vi "Unescape JSON String.vi"(11 "escaped string":string) -> (3 "regular string":string)   [LabVIEW 2020, in "Multi Error Cluster.lvlib"]
doc: "Convert an escaped JSON stringh into the originally supplied string. This allows a name to contain a /, '\", \\, or a control character."
uses:
  <vilib>/MultiError/TokenizeJSON/Multi Error Cluster.lvlib
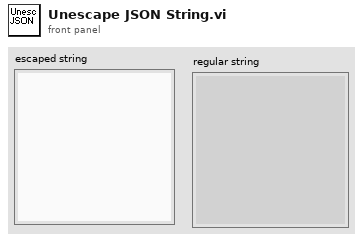
[diagram p1: front panel]
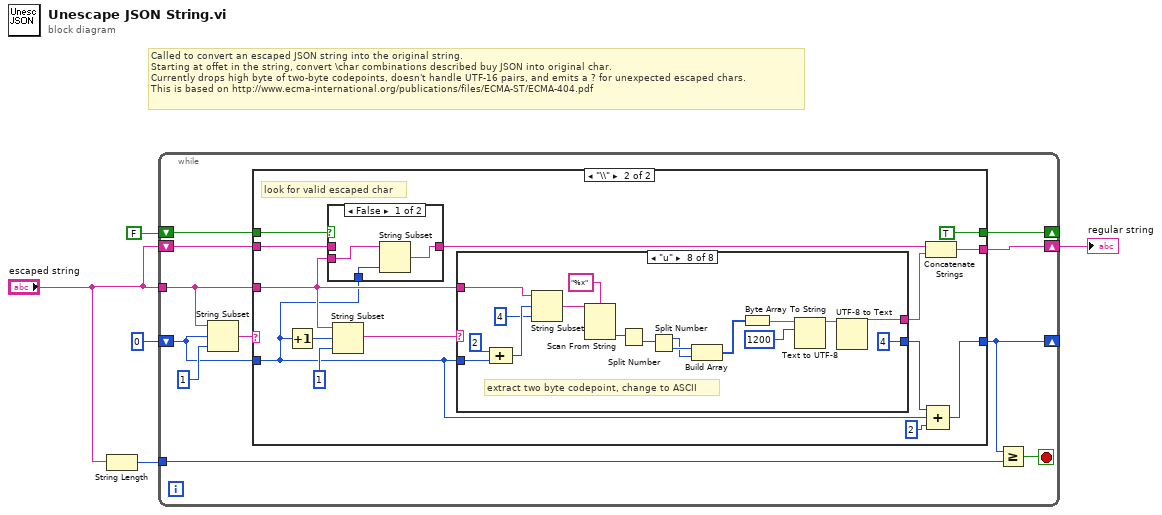
[diagram p0: block diagram]
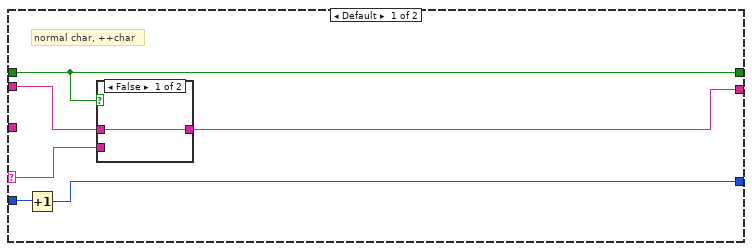
[diagram p2: hidden frame]
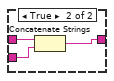
[diagram p3: hidden frame]
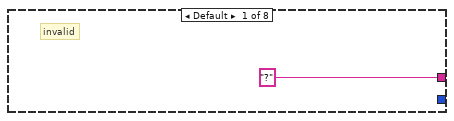
[diagram p5: hidden frame]
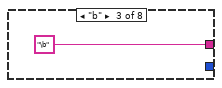
[diagram p7: hidden frame]
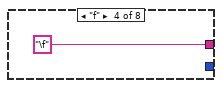
[diagram p8: hidden frame]
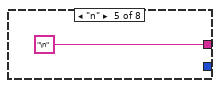
[diagram p9: hidden frame]
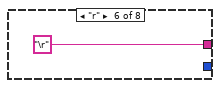
[diagram p10: hidden frame]
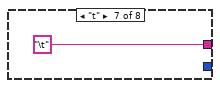
[diagram p11: hidden frame]
diagram:
  # "Called to convert an escaped JSON string into the original string.\nStarting at offet in the string, convert \\char combinations described buy JSON into original char.\nCurrently drops high byte of two-byte codepoints, doesn't handle UTF-16 pairs, and emits a ? for unexpected escaped chars.\nThis is based on http://www.ecma-international.org/publications/files/ECMA-ST/ECMA-404.pdf"
  n1 = String Length(string="escaped string") -> (length=w1:i32)
  n2 = while {
    tunnel: "escaped string" -> [w16]
    shift-right: [w6] -> _
    shift-left: 0 ("offset") -> [w8]
    shift-right: [w10] -> w2
    shift-left: "escaped string" -> [w13]
    shift-right: [w11] -> _
    shift-left: FALSE -> [w12]
    tunnel: w1 -> [w9]
    stop <- w7 stop-if-true
    n3 = String Subset(string=w16, offset (0)=w8, length (rest)=1) -> (substring=w14:string)
    n4 = case shown="\"\\\\\"" w14 {
      selector: w14 -> [w18 _]
      tunnel: w8 -> [w22 w32]
      tunnel: [w21 w27] -> w6
      tunnel: w16 -> [_ w33]
      tunnel: w13 -> [w19 w34]
      tunnel: w12 -> [w20 w35]
      tunnel: [w20 TRUE] -> w11
      tunnel: [w17 w29] -> w10
      frame Default {
        # "normal char, ++char"
        n5 = Increment(x=w22) -> (x+1=w21:i32)
        n6 = case shown="False" w20 {
          tunnel: w19 -> [w23 w26]
          tunnel: [w23 w24] -> w17
          tunnel: w18 -> [_ w25]
          frame False {
          }
          frame True {
            n7 = Concatenate Strings(w26, w25) -> (w24:string)
          }
        }
      }
      frame "\\" {
        # "look for valid escaped char"
        n8 = Increment(x=w32) -> (x+1=w40:i32)
        n9 = case shown="False" w35 {
          tunnel: w34 -> [_ w44]
          tunnel: [w41 w44] -> w31
          tunnel: w33 -> [w43 _]
          tunnel: w32 -> [w42 _]
          frame False {
            n10 = String Subset(string=w43, length (rest)=w42) -> (substring=w41:string)  [unwired: 1 in]
          }
          frame True {
          }
        }
        n11 = String Subset(string=w33, offset (0)=w40, length (rest)=1) -> (substring=w38:string)
        n12 = case shown="\"u\"" w38 {
          selector: w38 -> [_ w46 _ _ _ _ _ _]
          tunnel: w32 -> [_ _ _ _ _ _ _ w66]
          tunnel: [_ _ _ _ _ _ _ 4] -> w28
          tunnel: ["?" w46 "\b" "\f" "\n" "\r" "\t" w52] -> w30
          tunnel: w33 -> [_ _ _ _ _ _ _ w67]
          frame Default {
            # "invalid"
          }
          frame "\"", "/", "\\" {
          }
          frame "b" {
          }
          frame "f" {
          }
          frame "n" {
          }
          frame "r" {
          }
          frame "t" {
          }
          frame "u" {
            # "extract two byte codepoint, change to ASCII"
            n13 = Compound Arithmetic op=ADD(2, w66) -> (w64:i32)
            n14 = String Subset(string=w67, offset (0)=w64, length (rest)=4) -> (substring=w62:string)
            n15 = Scan From String(format string="%x", input string=w62) -> (output 1=w60:u32)  [unwired: 3 in, 3 out]
            n16 = Split Number(x=w60) -> (lo(x)=w59:u16)  [unwired: 1 out]
            n17 = Split Number(x=w59) -> (hi(x)=w56:u8, lo(x)=w58:u8)
            n18 = Build Array(w58, w56) -> (w57:u8[])
            n19 = Byte Array To String(unsigned byte array=w57) -> (string=w53:string)
            n20 = Text to UTF-8(10:1200 ("from encoding/code page (system default=-1)"), 11:w53) -> (3:w55:string)  [unwired: 1 in, 1 out]
            n21 = UTF-8 to Text(11:w55) -> (3:w52:string)  [unwired: 2 in, 1 out]
          }
        }
        n22 = Concatenate Strings(w31, w30) -> (w29:string)
        n23 = Compound Arithmetic op=ADD(w28, w32, 2) -> (w27:i32)
      }
    }
    n24 = Greater Or Equal?(x=w6, y=w9) -> (x >= y?=w7:bool)
  }
  "regular string" <- w2
